vi "Select Autocomplete Match.vi"(7 "String in":refnum<vi>, 9 "Match Index":i32, 11 "Autocomplete State in":T1) -> (3 "Autocomplete State out":T1)   [LabVIEW 2020, in "Output Sequencer.lvlib" / "Settings UI.lvclass"]
uses:
  Settings UI.lvclass
  Types/Autocomplete State.ctl
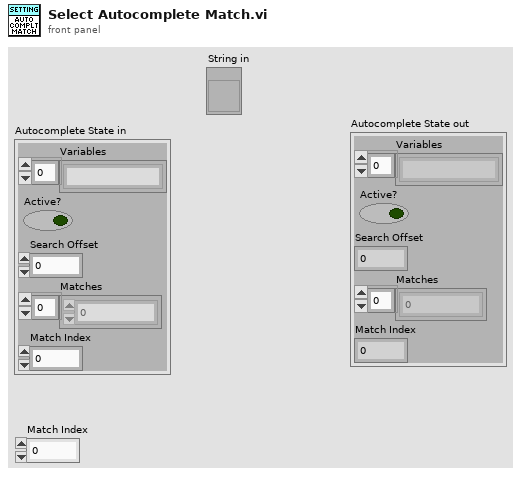
[diagram p1: front panel]
types:
  T1 = typedef "Output Sequencer.lvlib/Settings UI.lvclass/Autocomplete State.ctl" = cluster{"Variables":string[], "Active?":bool, "Search Offset":i32, "Matches":i32[], "Match Index":i32}
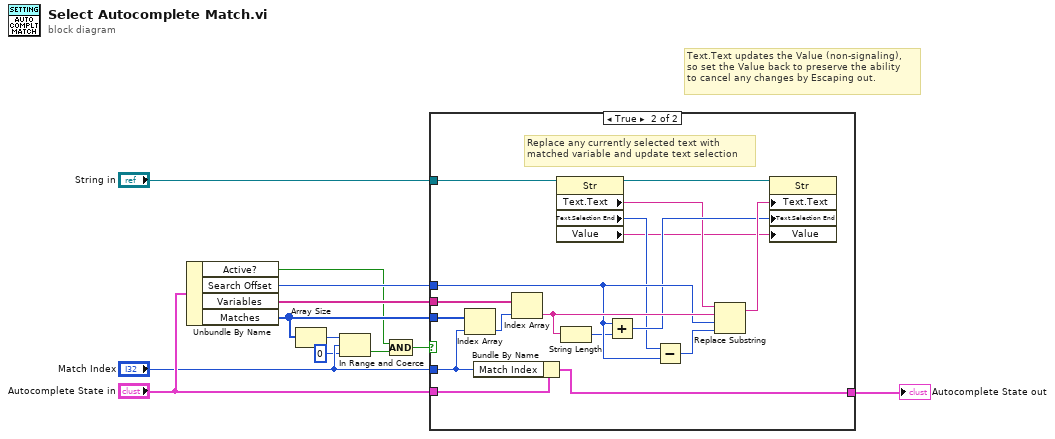
[diagram p0: block diagram]
diagram:
  # "Text.Text updates the Value (non-signaling),\nso set the Value back to preserve the ability\nto cancel any changes by Escaping out."
  n1 = Unbundle By Name("Autocomplete State in") -> ("Active?"=w1:bool, "Search Offset"=w7:i32, "Variables"=w8:string[], "Matches"=w6:i32[])
  n2 = Array Size(array=w6) -> (size(s)=w4:i32)
  n3 = In Range and Coerce(upper limit=w4, x="Match Index", lower limit=0) -> (In Range?=w3:bool)  [unwired: 1 out]
  n4 = Compound Arithmetic op=AND(w1, w3) -> (w5:bool)
  n5 = case shown="True" w5 {
    tunnel: "Autocomplete State in" -> [w13 w22]
    tunnel: [w13 w20] -> w11
    tunnel: w7 -> [_ w26]
    tunnel: w8 -> [_ w30]
    tunnel: "Match Index" -> [_ w21]
    tunnel: "String in" -> [_ w24]
    tunnel: w6 -> [_ w23]
    frame False {
      # "Autocomplete isn't active, or the\ndesired match index isn't valid."
    }
    frame True {
      # "Replace any currently selected text with\nmatched variable and update text selection"
      n6 = Index Array(array=w23, index=w21) -> (element=w29:i32)
      n7 = Bundle By Name(cluster=w22, "Match Index"=w21) -> (w20:T1)
      n8 = Index Array(array=w30, index=w29) -> (element=w28:string)
      n9 = property class="Str"(reference=w24) -> (reference out=w25:refnum<vi>, "Text.Text"=w18:string, "Text.Selection End"=w17:u32, "Value"=w14:string)  [unwired: 1 in, 1 out]
      n10 = String Length(string=w28) -> (length=w15:i32)
      n11 = Add(x=w26, y=w15) -> (x+y=w19:i32)
      n12 = Subtract(x=w17, y=w26) -> (x-y=w16:u32)
      n13 = Replace Substring(2:w16, 3:w26, 4:w28, 5:w18) -> (1:w27:string)  [unwired: 1 out]
      n14 = property on="Property Node" class="Str"(reference=w25, "Text.Text"=w27, "Text.Selection End"=w19, "Value"=w14) -> ()  [unwired: 1 in, 2 out]
    }
  }
  "Autocomplete State out" <- w11
